vi "RichToFlatnixnet_grpc_LinDiagnosticScheduleChangeRequest.vi"(5 "OutputClusterType":T1, 11 "InputCluster":T3) -> (3 "OutputCluster":T1)   [LabVIEW 2025, in "xnet-grpc_client.lvlib"]
uses:
  xnet-grpc_client.lvlib
  nixnet_grpc_LinDiagnosticScheduleChangeRequest.ctl
  nixnet_grpc_LinDiagnosticScheduleChangeRequest_schedule_enum/nixnet_grpc_LinDiagnosticScheduleChangeRequest_schedule_enum.lvclass
  nixnet_grpc_LinDiagnosticScheduleChangeRequest_Flat.ctl
  nixnet_grpc_LinDiagnosticSchedule.ctl
  nixnet_grpc_LinDiagnosticScheduleChangeRequest_schedule_enum/nixnet_grpc_LinDiagnosticScheduleChangeRequest_schedule_enum.lvclass/nixnet_grpc_LinDiagnosticScheduleChangeRequest_schedule_enum.ctl
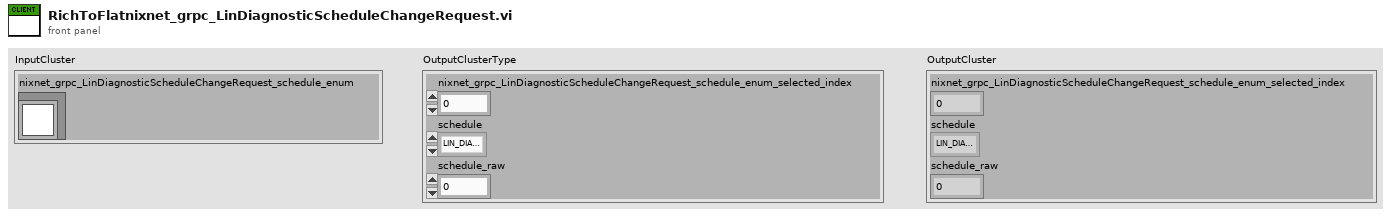
[diagram p1: front panel]
types:
  T1 = typedef "xnet-grpc_client.lvlib/nixnet_grpc_LinDiagnosticScheduleChangeRequest_Flat.ctl" = cluster{"nixnet_grpc_LinDiagnosticScheduleChangeRequest_schedule_enum_selected_index":i32, "schedule":T2, "schedule_raw":u32}
  T2 = typedef "xnet-grpc_client.lvlib/nixnet_grpc_LinDiagnosticSchedule.ctl" = enum32{"LIN_DIAGNOSTIC_SCHEDULE_NULL", "LIN_DIAGNOSTIC_SCHEDULE_MASTER_REQ", "LIN_DIAGNOSTIC_SCHEDULE_SLAVE_RESP"}
  T3 = typedef "xnet-grpc_client.lvlib/nixnet_grpc_LinDiagnosticScheduleChangeRequest.ctl" = cluster{"nixnet_grpc_LinDiagnosticScheduleChangeRequest_schedule_enum":refnum<class "nixnet_grpc_LinDiagnosticScheduleChangeRequest_schedule_enum.lvclass">}
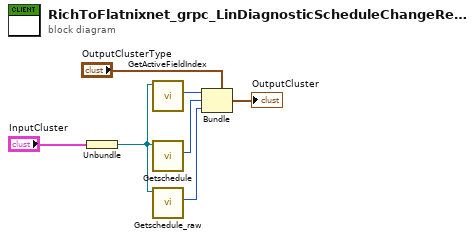
[diagram p0: block diagram]
diagram:
  n1 = Unbundle "Unbundle"("InputCluster") -> ("nixnet_grpc_LinDiagnosticScheduleChangeRequest_schedule_enum"=w4:refnum<class "nixnet_grpc_LinDiagnosticScheduleChangeRequest_schedule_enum.lvclass">)
  n2 = call "GetActiveFieldIndex.vi"("OneOfTemplate in"=w4) -> ("Active Field Index"=w3:i32)  [unwired: 8 in, 2 out]
  n3 = call "Getschedule.vi"("OneOfTemplate in"=w4) -> ("Get_Val"=w2:T2)  [unwired: 8 in, 2 out]
  n4 = call "Getschedule_raw.vi"("OneOfTemplate in"=w4) -> ("Get_Val"=w1:u32)  [unwired: 8 in, 2 out]
  n5 = Bundle "Bundle"(cluster="OutputClusterType", "nixnet_grpc_LinDiagnosticScheduleChangeRequest_schedule_enum_selected_index"=w3, "schedule"=w2, "schedule_raw"=w1) -> (→"OutputCluster":T1)
